vi "New Input.vi"(8 "error in (no error)":errorcluster, 11 "Descriptor":string) -> (0 "error out":errorcluster, 3 "input out":refnum<class "Input.lvclass">)   [LabVIEW 2015, in "Input.lvclass"]
uses:
  Input.lvclass
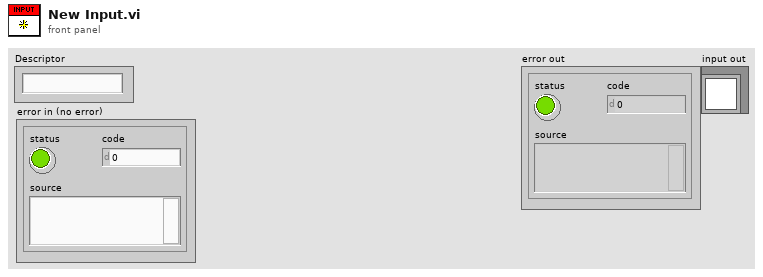
[diagram p1: front panel]
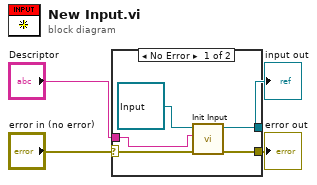
[diagram p0: block diagram]
diagram:
  n1 = case shown="No Error" "error in (no error)" {
    selector: "error in (no error)" -> [w9 w10]
    tunnel: "Descriptor" -> [w8 _]
    tunnel: [w6 w10] -> w3
    tunnel: [w7 _] -> w1
    frame No Error {
      n2 = call-dynamic "Init Input.vi"("error in (no error)"=w9, "Descriptor"=w8, "input in"=refnum<class "Input.lvclass"> refnum ("Input.lvclass")) -> ("error out"=w6:errorcluster, "input out"=w7:refnum<class "Input.lvclass">)  [unwired: 7 in]
    }
    frame Error {
    }
  }
  "error out" <- w3
  "input out" <- w1
